vi "Fit Sinusoidal Gain.vi"(4 "Trace Select":i32 min=0 max=1000, 6 "reference 4":refnum<vi>, 7 "Cluster in":T1={"Impulse Positions"=[], "Data File"={"Data Channels"=[], "Sample Rate"=0, "Channel List"=[]}, "desaccading parameters"={"Tolerance"=0, "Acc Range"=0.0, "Sample Rate"=0, "Impulse Plane 2"=enum."Other", "Impulse dir"=FALSE}, "Stimulus"=[], "Response"=[], "Fitted Curves"=[], "Sinusoidal Fit Controls"={"Sinusoidal Response"={"Offset"=0.0, "Gain"=0.0, "Phase"=0.0, "Freq"=0.0}, "Sinusoidal Stimulus"={"Offset"=-0.1762531244084861, "Gain"=54.01231242273056, "Phase"=48.997269246957444, "Freq"=8.0}, "Stimulus\nFrequency"=8.0, "Stat."=enum."Ind. Traces", "Use Values Above to Calculate Gains"=FALSE, "Automatically Calculate \nStimulus Frequency"=FALSE, "Gain and Phase"={"Gain"=0.0, "Gain SD"=0.0, "Phase"=0.0, "Phase SD"=0.0}}, "Transient Gains"={"Line Fit Response"={"Offset"=0.0, "Slope"=0.0}, "Stimulus Equation"="", "Reponse Equation"="", "Gv"=0.0, "Ga"=0.0, "Line Fit Stimulus"={"Offset"=0.0, "Slope"=0.0}, "Ga Window (early)"=0, "Gv Window"=0, "Latency (ms)"=0.0, "Stim.Onset"=0.0, "TH/#SDs 2"=0.0, "Response Onset"=0.0, "Snap Cursor"=0, "Latency"=0, "Poly. Window"=0, "Ord."=0, "BIC"=0.0, "Poly Equation"="", "Gv SD"=0.0, "Ga SD"=0.0, "Ga Stat."=0, "Mirror"=FALSE, "MSE"=0.0, "Gv Stat."=0, "Ga 2"=0.0, "Ga SD 2"=0.0, "Ga Window  (late)"=0, "Ga Stat. 2"=0, "GV desaccading"=FALSE, "GA2 desaccading"=FALSE, "GA1 desaccading"=FALSE, "Line Fit Response 2"={"Offset"=0.0, "Slope"=0.0}, "Stimulus Equation 2"="", "Reponse Equation 2"="", "Line Fit Stimulus 2"={"Offset"=0.0, "Slope"=0.0}, "Show Line Fit Parameters "=FALSE, "Gv Line Fit Stimulus"={"Offset"=0.0, "Slope"=0.0}, "Gv Line Fit Response"={"Offset"=0.0, "Slope"=0.0}, "Latency window"=0, "Latency Stat."=0, "Line Fit Res Latency"={"Offset"=0.0, "Slope"=0.0}, "Stim Eq Latency"="", "Resp Eq Latency"="", "Line Fit Stim Latency"={"Offset"=0.0, "Slope"=0.0}, "GA Line active"=0}, "Gv Line Fit Stimulus"={"Offset"=0.0, "Slope"=0.0}, "Gv Line Fit Response"={"Offset"=0.0, "Slope"=0.0}, "Fit Calculated"=FALSE, "Excel"={"Excel._Application"=refnum, "Use Excel"=FALSE, "Worksheet SINE"=refnum, "Row SINE"=0, "Worksheet TRANS"=refnum, "Row TRANS"=0}, "desacc "={"Threshold 1 [Acc]"=0.0, "Threshold 2 [% of TH1]"=0, "tolerance"=0, "Search WD "=0.0, " always use TH2"=FALSE, "Range"=0.0, "Max time"=0.0, "Min time"=0.0, "Velocity Threshold"=0}, "Impulse Data"=refnum, "Impulse Manager"=refnum, "Graph Manager"=refnum, "Sine Fit"=[], "Excel Logger"=refnum, "Halfwave Fit Display"=refnum, "Mean Fit"=refnum} {"Sinusoidal Fit Controls"."Gain and Phase"."Phase SD" format="%.1f"; "Sinusoidal Fit Controls"."Gain and Phase"."Phase" format="%.1f"; "Sinusoidal Fit Controls"."Gain and Phase"."Gain SD" format="%.2f"; "Sinusoidal Fit Controls"."Gain and Phase"."Gain" format="%.2f"; "Sinusoidal Fit Controls"."Stimulus\nFrequency" format="%.2f"; "Sinusoidal Fit Controls"."Sinusoidal Stimulus"."Freq" format="%#.2f"; "Sinusoidal Fit Controls"."Sinusoidal Stimulus"."Offset" format="%.3f"; "Sinusoidal Fit Controls"."Sinusoidal Stimulus"."Gain" format="%.2f"; "Sinusoidal Fit Controls"."Sinusoidal Stimulus"."Phase" format="%.1f"; "Sinusoidal Fit Controls"."Sinusoidal Response"."Freq" format="%#.2f"; "Sinusoidal Fit Controls"."Sinusoidal Response"."Offset" format="%.3f"; "Sinusoidal Fit Controls"."Sinusoidal Response"."Gain" format="%.2f"; "Sinusoidal Fit Controls"."Sinusoidal Response"."Phase" format="%.1f"}, 9 "reference 3":refnum<vi>, 10 "reference in":refnum<vi>, 11 "Array in":refnum<vi>) -> (3 "Cluster out":T1={"Impulse Positions"=[], "Data File"={"Data Channels"=[], "Sample Rate"=0, "Channel List"=[]}, "desaccading parameters"={"Tolerance"=0, "Acc Range"=0.0, "Sample Rate"=0, "Impulse Plane 2"=enum."Other", "Impulse dir"=FALSE}, "Stimulus"=[], "Response"=[], "Fitted Curves"=[], "Sinusoidal Fit Controls"={"Sinusoidal Response"={"Offset"=0.0, "Gain"=0.0, "Phase"=0.0, "Freq"=0.0}, "Sinusoidal Stimulus"={"Offset"=-0.1762531244084861, "Gain"=54.01231242273056, "Phase"=48.997269246957444, "Freq"=8.0}, "Stimulus\nFrequency"=8.0, "Stat."=enum."Ind. Traces", "Use Values Above to Calculate Gains"=FALSE, "Automatically Calculate \nStimulus Frequency"=FALSE, "Gain and Phase"={"Gain"=0.0, "Gain SD"=0.0, "Phase"=0.0, "Phase SD"=0.0}}, "Transient Gains"={"Line Fit Response"={"Offset"=0.0, "Slope"=0.0}, "Stimulus Equation"="", "Reponse Equation"="", "Gv"=0.0, "Ga"=0.0, "Line Fit Stimulus"={"Offset"=0.0, "Slope"=0.0}, "Ga Window (early)"=0, "Gv Window"=0, "Latency (ms)"=0.0, "Stim.Onset"=0.0, "TH/#SDs 2"=0.0, "Response Onset"=0.0, "Snap Cursor"=0, "Latency"=0, "Poly. Window"=0, "Ord."=0, "BIC"=0.0, "Poly Equation"="", "Gv SD"=0.0, "Ga SD"=0.0, "Ga Stat."=0, "Mirror"=FALSE, "MSE"=0.0, "Gv Stat."=0, "Ga 2"=0.0, "Ga SD 2"=0.0, "Ga Window  (late)"=0, "Ga Stat. 2"=0, "GV desaccading"=FALSE, "GA2 desaccading"=FALSE, "GA1 desaccading"=FALSE, "Line Fit Response 2"={"Offset"=0.0, "Slope"=0.0}, "Stimulus Equation 2"="", "Reponse Equation 2"="", "Line Fit Stimulus 2"={"Offset"=0.0, "Slope"=0.0}, "Show Line Fit Parameters "=FALSE, "Gv Line Fit Stimulus"={"Offset"=0.0, "Slope"=0.0}, "Gv Line Fit Response"={"Offset"=0.0, "Slope"=0.0}, "Latency window"=0, "Latency Stat."=0, "Line Fit Res Latency"={"Offset"=0.0, "Slope"=0.0}, "Stim Eq Latency"="", "Resp Eq Latency"="", "Line Fit Stim Latency"={"Offset"=0.0, "Slope"=0.0}, "GA Line active"=0}, "Gv Line Fit Stimulus"={"Offset"=0.0, "Slope"=0.0}, "Gv Line Fit Response"={"Offset"=0.0, "Slope"=0.0}, "Fit Calculated"=FALSE, "Excel"={"Excel._Application"=refnum, "Use Excel"=FALSE, "Worksheet SINE"=refnum, "Row SINE"=0, "Worksheet TRANS"=refnum, "Row TRANS"=0}, "desacc "={"Threshold 1 [Acc]"=0.0, "Threshold 2 [% of TH1]"=0, "tolerance"=0, "Search WD "=0.0, " always use TH2"=FALSE, "Range"=0.0, "Max time"=0.0, "Min time"=0.0, "Velocity Threshold"=0}, "Impulse Data"=refnum, "Impulse Manager"=refnum, "Graph Manager"=refnum, "Sine Fit"=[], "Excel Logger"=refnum, "Halfwave Fit Display"=refnum, "Mean Fit"=refnum} {"Sinusoidal Fit Controls"."Gain and Phase"."Phase SD" format="%.1f"; "Sinusoidal Fit Controls"."Gain and Phase"."Phase" format="%.1f"; "Sinusoidal Fit Controls"."Gain and Phase"."Gain SD" format="%.2f"; "Sinusoidal Fit Controls"."Gain and Phase"."Gain" format="%.2f"; "Sinusoidal Fit Controls"."Stimulus\nFrequency" format="%.2f"; "Sinusoidal Fit Controls"."Sinusoidal Stimulus"."Freq" format="%#.2f"; "Sinusoidal Fit Controls"."Sinusoidal Stimulus"."Offset" format="%.3f"; "Sinusoidal Fit Controls"."Sinusoidal Stimulus"."Gain" format="%.2f"; "Sinusoidal Fit Controls"."Sinusoidal Stimulus"."Phase" format="%.1f"; "Sinusoidal Fit Controls"."Sinusoidal Response"."Freq" format="%#.2f"; "Sinusoidal Fit Controls"."Sinusoidal Response"."Offset" format="%.3f"; "Sinusoidal Fit Controls"."Sinusoidal Response"."Gain" format="%.2f"; "Sinusoidal Fit Controls"."Sinusoidal Response"."Phase" format="%.1f"})   [LabVIEW 2013]
uses:
  comm/nan operations/nan operations.lvlib
  <vilib>/Analysis/NI_AALPro.lvlib
  comm/impulse/impulse functions.lvlib
  comm/stats/stats.lvlib
  <vilib>/Analysis/NI_AALBase.lvlib
  <vilib>/Analysis/baseanly.llb/Mean (DBL).vi
  <vilib>/Analysis/1siggen.llb/Ramp Pattern by Samples.vi
  core/Classes/Sinusoidal Fit/Sinusoidal Fit.lvclass
  Polimorphic Gain and Phase VIs/Cluster Gain and Phase.vi
  Polimorphic Gain and Phase VIs/Mean Gain and Phase.vi
  Typedef_StatisticType.ctl
  Typedef - Gain and Phase.ctl
  Typedef - Sinusoidal Fit Coefficients.ctl
  Typedef - Data Analyser Main Cluster.ctl
  Typedef - Sinusoidal Fit Controls.ctl
  core/Classes/Impulse Data/Impulse Data.lvclass
  core/Classes/Impulse Manager/Impulse Manager.lvclass
  core/Classes/Impulse Data/Instance handle.ctl
  core/Classes/Graph Manager/Graph Manager.lvclass
  core/Classes/Excel Logger/Excel Logger.lvclass
  core/Classes/Fit Displays/Halfwave Fit Display/Halfwave Fit Display.lvclass
  core/Classes/Mean Fit/Mean Fit.lvclass
panel:
  # "Gain:"
  # "+/-"
  # "Phase:"
  # "+/-"
  # "Gain:"
  # "+/-"
  # "Phase:"
  # "+/-"
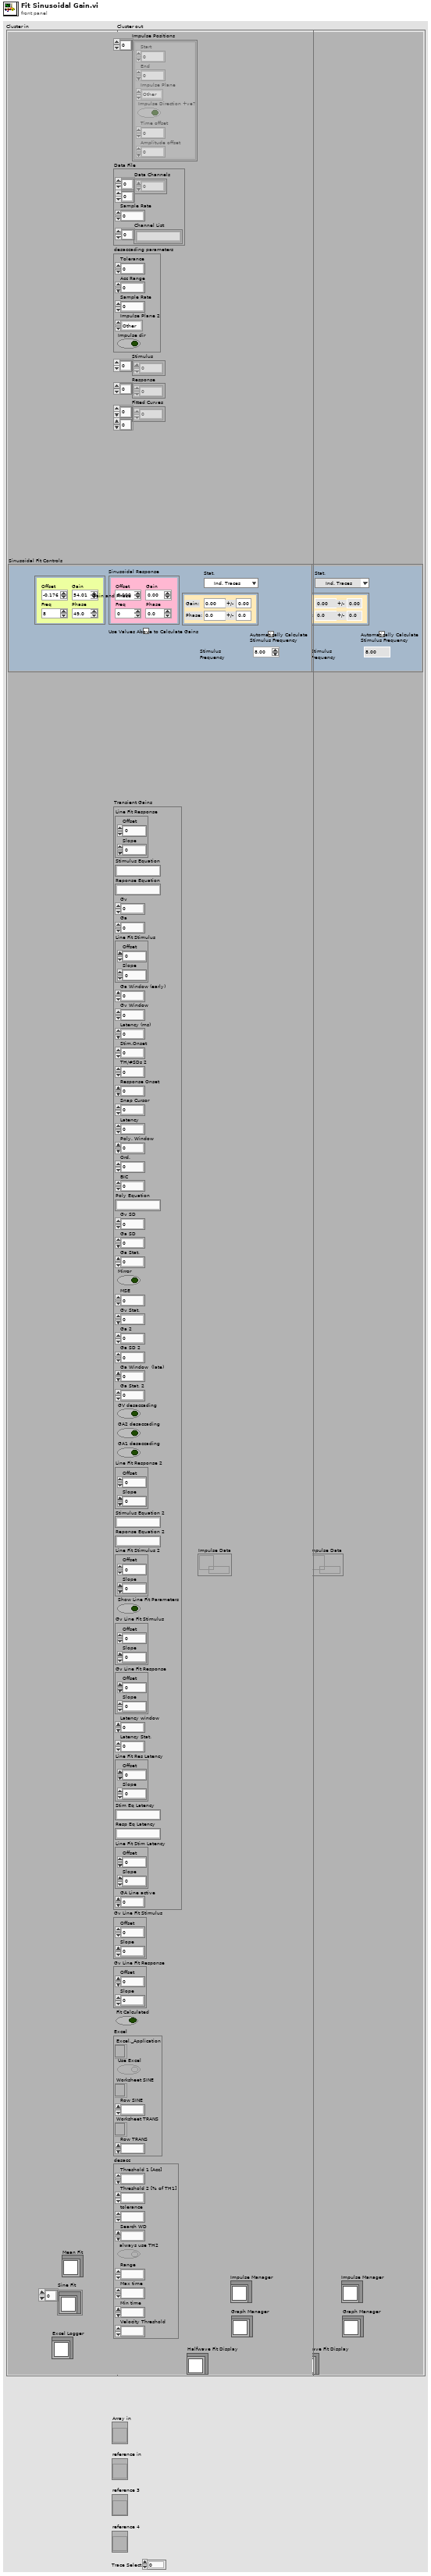
[diagram p1: front panel]
types:
  T1 = typedef "Typedef - Data Analyser Main Cluster.ctl" = cluster{"Impulse Positions":cluster{"Start":i32, "End":i32, "Impulse Plane":enum16{"Other", "Yaw", "Pitch", "Roll", "LARP", "RALP"}, "Impulse Direction +ve?":bool, "Time offset":i32, "Amplitude offset":dbl}[], "Data File":cluster{"Data Channels":dbl[][], "Sample Rate":i32, "Channel List":string[]}, "desaccading parameters":cluster{"Tolerance":i32, "Acc Range":dbl, "Sample Rate":i32, "Impulse Plane 2":enum16{"Other", "Yaw", "Pitch", "Roll", "LARP", "RALP"}, "Impulse dir":bool}, "Stimulus":dbl[], "Response":dbl[], "Fitted Curves":dbl[][], "Sinusoidal Fit Controls":T2, "Transient Gains":cluster{"Line Fit Response":cluster{"Offset":dbl, "Slope":dbl}, "Stimulus Equation":string, "Reponse Equation":string, "Gv":dbl, "Ga":dbl, "Line Fit Stimulus":cluster{"Offset":dbl, "Slope":dbl}, "Ga Window (early)":u16, "Gv Window":u16, "Latency (ms)":dbl, "Stim.Onset":dbl, "TH/#SDs 2":dbl, "Response Onset":dbl, "Snap Cursor":u16, "Latency":u16, "Poly. Window":u16, "Ord.":i32, "BIC":dbl, "Poly Equation":string, "Gv SD":dbl, "Ga SD":dbl, "Ga Stat.":u16, "Mirror":bool, "MSE":dbl, "Gv Stat.":u16, "Ga 2":dbl, "Ga SD 2":dbl, "Ga Window  (late)":u16, "Ga Stat. 2":u16, "GV desaccading":bool, "GA2 desaccading":bool, "GA1 desaccading":bool, "Line Fit Response 2":cluster{"Offset":dbl, "Slope":dbl}, "Stimulus Equation 2":string, "Reponse Equation 2":string, "Line Fit Stimulus 2":cluster{"Offset":dbl, "Slope":dbl}, "Show Line Fit Parameters ":bool, "Gv Line Fit Stimulus":cluster{"Offset":dbl, "Slope":dbl}, "Gv Line Fit Response":cluster{"Offset":dbl, "Slope":dbl}, "Latency window":u16, "Latency Stat.":u16, "Line Fit Res Latency":cluster{"Offset":dbl, "Slope":dbl}, "Stim Eq Latency":string, "Resp Eq Latency":string, "Line Fit Stim Latency":cluster{"Offset":dbl, "Slope":dbl}, "GA Line active":i32}, "Gv Line Fit Stimulus":cluster{"Offset":dbl, "Slope":dbl}, "Gv Line Fit Response":cluster{"Offset":dbl, "Slope":dbl}, "Fit Calculated":bool, "Excel":cluster{"Excel._Application":refnum<k7>, "Use Excel":bool, "Worksheet SINE":refnum<k7>, "Row SINE":i32, "Worksheet TRANS":refnum<k7>, "Row TRANS":i32}, "desacc ":cluster{"Threshold 1 [Acc]":dbl, "Threshold 2 [% of TH1]":i32, "tolerance":i32, "Search WD ":dbl, " always use TH2":bool, "Range":dbl, "Max time":dbl, "Min time":dbl, "Velocity Threshold":i32}, "Impulse Data":T6, "Impulse Manager":refnum<class "Impulse Manager.lvclass">, "Graph Manager":refnum<class "Graph Manager.lvclass">, "Sine Fit":refnum<class "Sinusoidal Fit.lvclass">[], "Excel Logger":refnum<class "Excel Logger.lvclass">, "Halfwave Fit Display":refnum<class "Halfwave Fit Display.lvclass">, "Mean Fit":refnum<class "Mean Fit.lvclass">}
  T2 = typedef "Typedef - Sinusoidal Fit Controls.ctl" = cluster{"Sinusoidal Response":T3, "Sinusoidal Stimulus":T3, "Stimulus\nFrequency":dbl, "Stat.":T4, "Use Values Above to Calculate Gains":bool, "Automatically Calculate \nStimulus Frequency":bool, "Gain and Phase":T5}
  T3 = typedef "Typedef - Sinusoidal Fit Coefficients.ctl" = cluster{"Offset":dbl, "Gain":dbl, "Phase":dbl, "Freq":dbl}
  T4 = typedef "Typedef_StatisticType.ctl" = enum16{"Mean Trace", "Ind. Traces"}
  T5 = typedef "Typedef - Gain and Phase.ctl" = cluster{"Gain":dbl, "Gain SD":dbl, "Phase":dbl, "Phase SD":dbl}
  T6 = typedef "Impulse Data.lvclass/Instance handle.ctl" = refnum<data-value>
  T7 = cluster{"Data Channels":dbl[][], "Sample Rate":i32, "Channel List":string[]}
  T8 = cluster{"Start":i32, "End":i32, "Impulse Plane":enum16{"Other", "Yaw", "Pitch", "Roll", "LARP", "RALP"}, "Impulse Direction +ve?":bool, "Time offset":i32, "Amplitude offset":dbl}[]
  T9 = enum16{"Other", "Yaw", "Pitch", "Roll", "LARP", "RALP"}
  T10 = cluster{"Threshold 1 [Acc]":dbl, "Threshold 2 [% of TH1]":i32, "tolerance":i32, "Search WD ":dbl, " always use TH2":bool, "Range":dbl, "Max time":dbl, "Min time":dbl, "Velocity Threshold":i32}
  T11 = typedef "core.lvlib/TD_Impulse Parameter.ctl" = cluster{"Color Box":u32, "Boolean":bool, "List 2":u16, "Boolean 2":bool, "Boolean 3":bool, "Offset":dbl, "Gain":dbl}[]
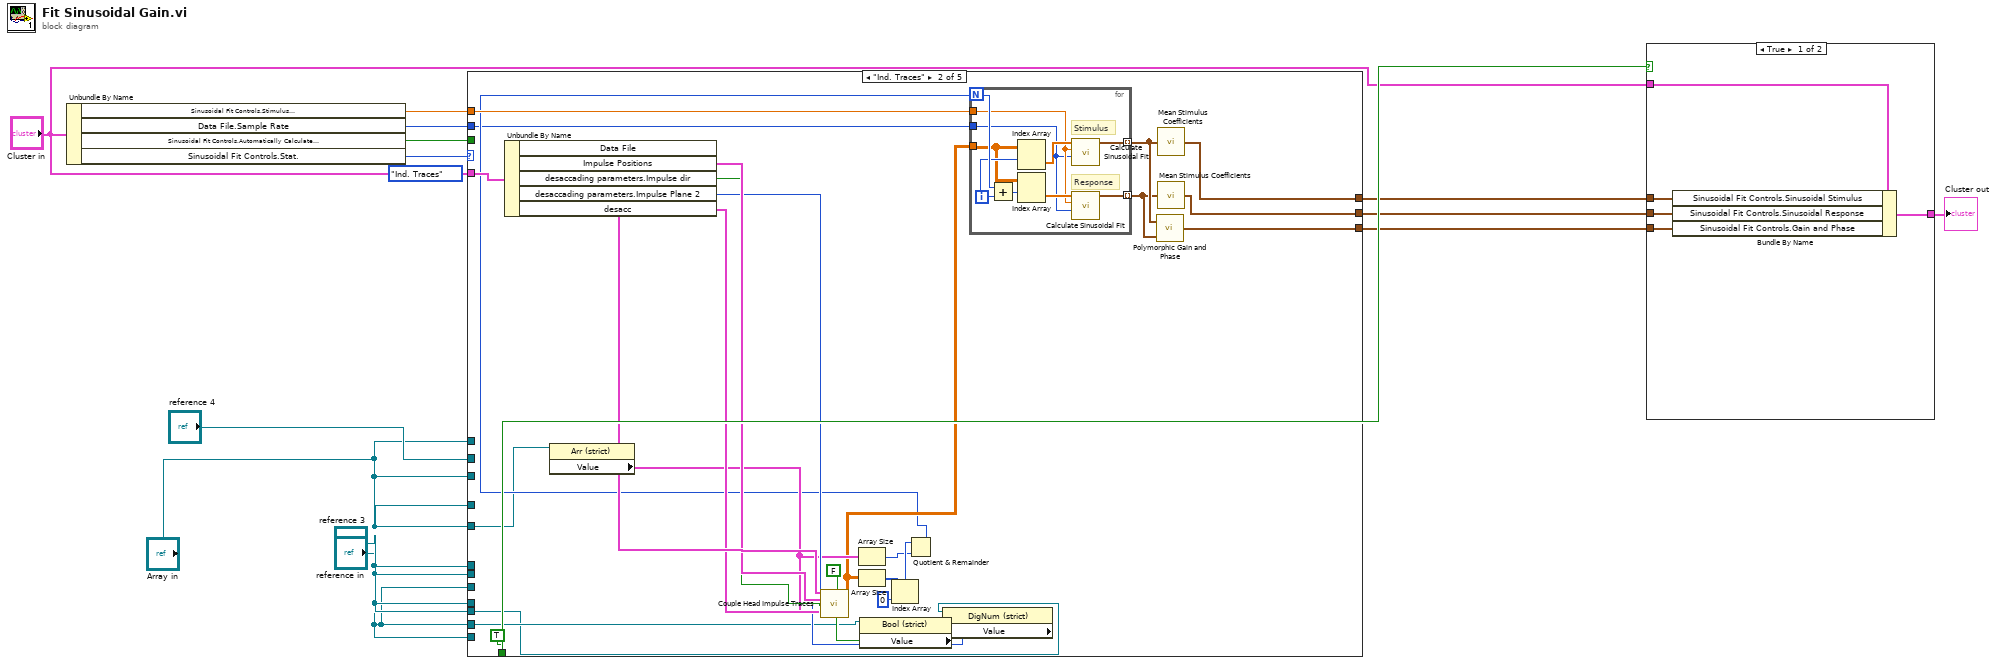
[diagram p0: block diagram]
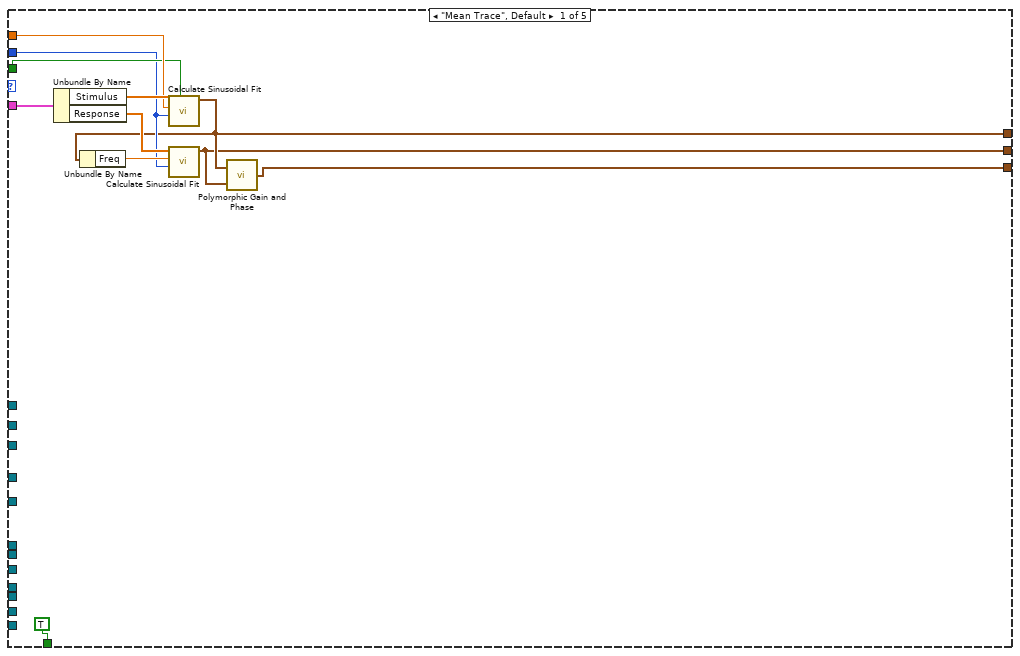
[diagram p2: hidden frame]
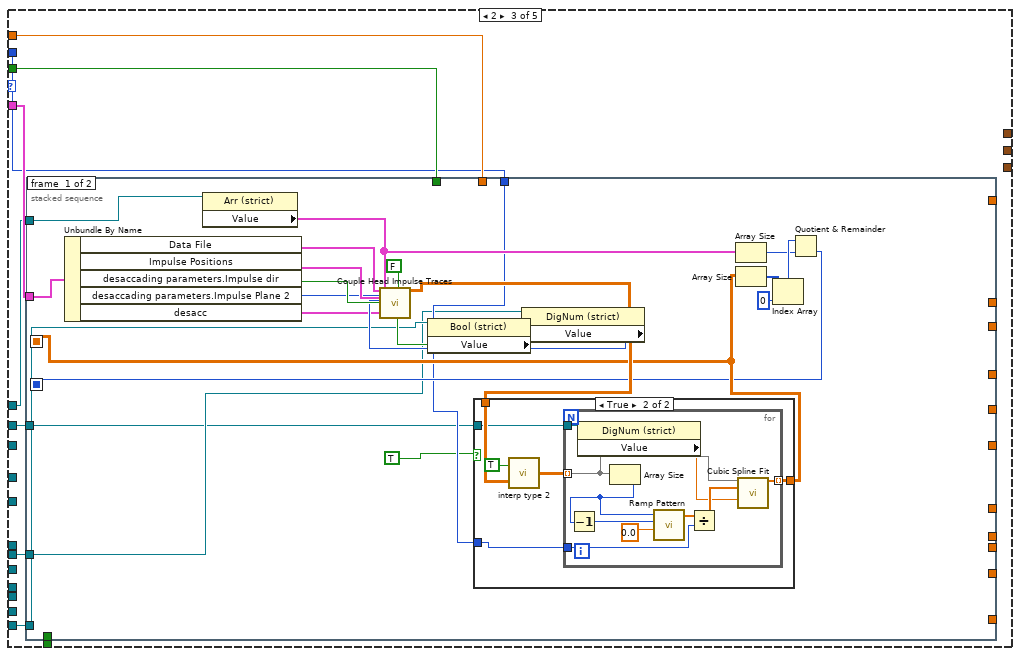
[diagram p3: hidden frame]
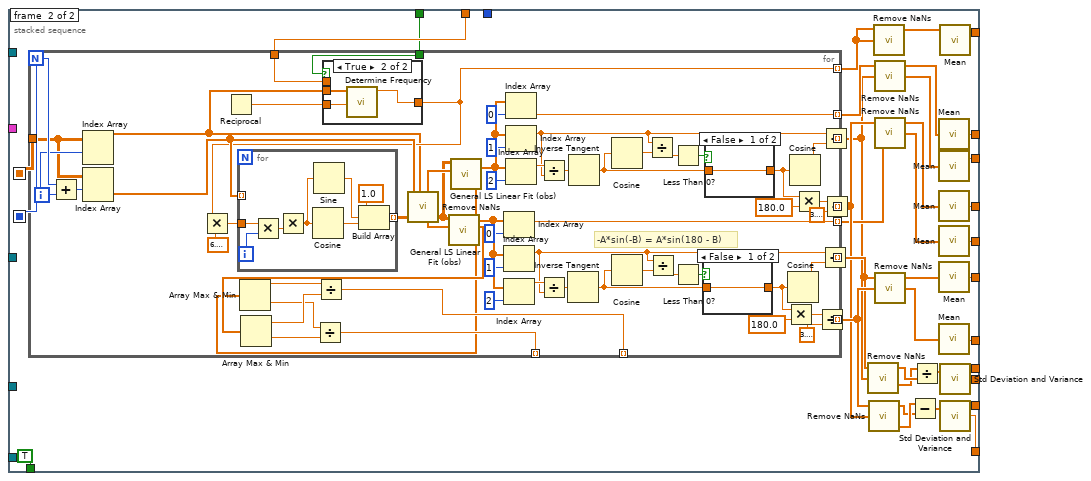
[diagram p5: hidden frame]
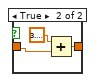
[diagram p7: hidden frame]
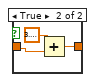
[diagram p8: hidden frame]
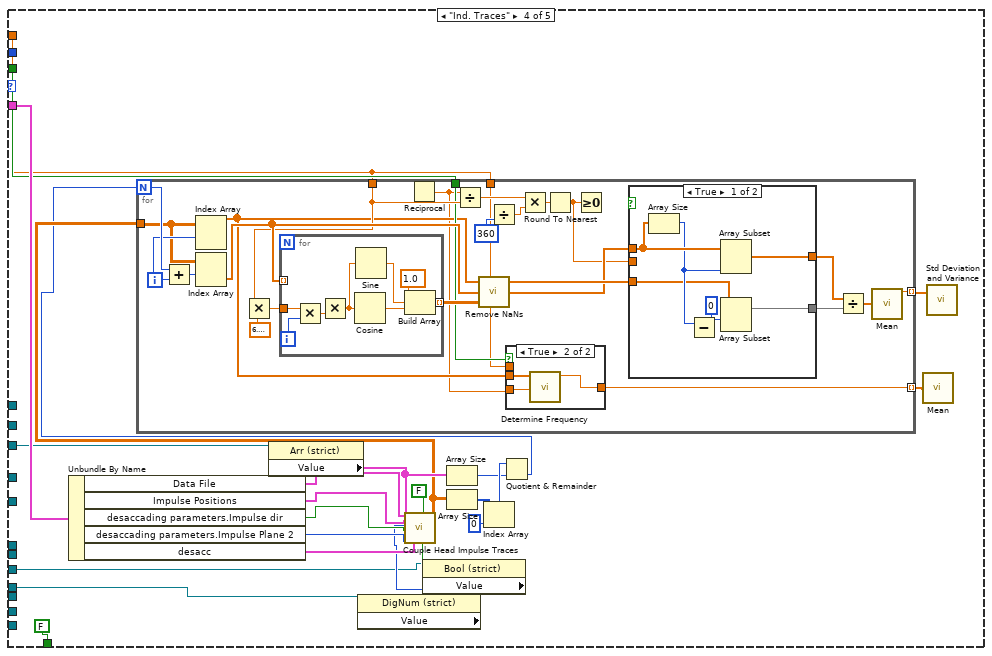
[diagram p9: hidden frame]
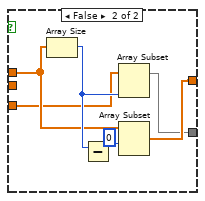
[diagram p11: hidden frame]
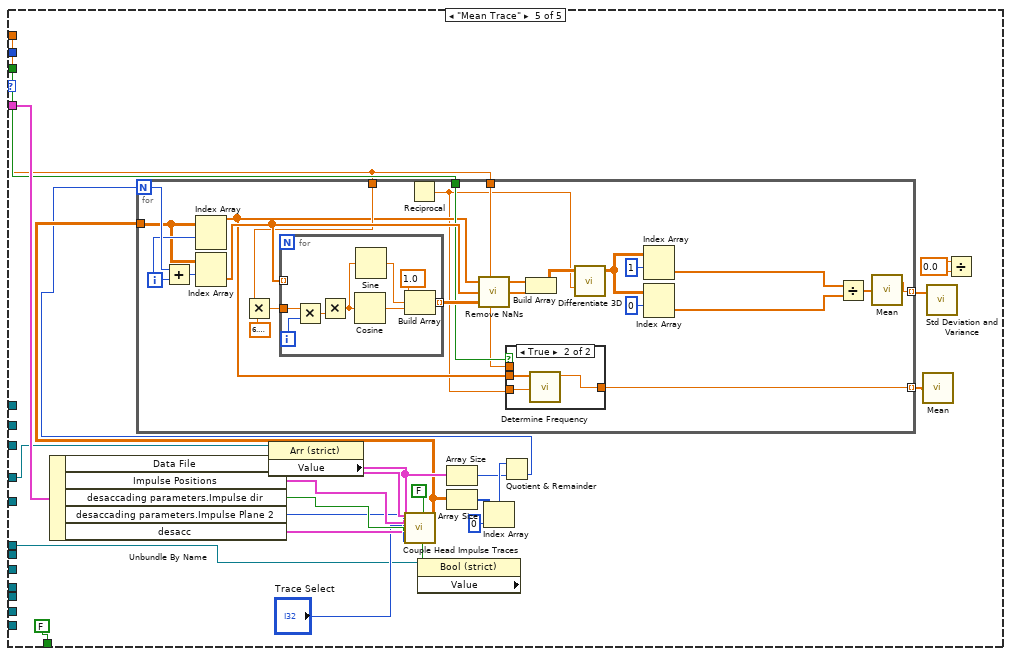
[diagram p12: hidden frame]
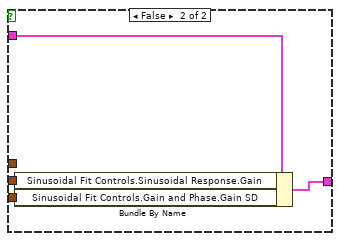
[diagram p14: hidden frame]
diagram:
  (unwired) Typedef_StatisticType."Ind. Traces" ("Sinusoidal Fit Controls.Stat.")
  n1 = Unbundle By Name("Cluster in") -> ("Sinusoidal Fit Controls.Stimulus\nFrequency"=w13:dbl, "Data File.Sample Rate"=w1:i32, "Sinusoidal Fit Controls.Automatically Calculate \nStimulus Frequency"=w14:bool, "Sinusoidal Fit Controls.Stat."=w10:T4)
  n2 = case shown="\"Ind. Traces\"" w10 {
    tunnel: w13 -> [w22 w52 w71 w236 w308]
    tunnel: "Cluster in" -> [w25 w40 w68 w242 w315]
    tunnel: [TRUE TRUE w70 FALSE FALSE] -> w12
    tunnel: w14 -> [w21 _ w69 w237 w309]
    tunnel: w1 -> [w18 w31 w67 _ _]
    tunnel: "Array in" -> [_ w34 _ _ _]
    tunnel: "reference in" -> [_ w33 _ _ _]
    tunnel: "reference 3" -> [_ w32 _ _ _]
    tunnel: "Array in" -> [_ _ w66 _ _]
    tunnel: "reference in" -> [_ _ w65 _ _]
    tunnel: "reference 3" -> [_ _ w64 _ _]
    tunnel: "reference 4" -> [_ _ w63 _ _]
    tunnel: "Array in" -> [_ _ _ w232 _]
    tunnel: "reference in" -> [_ _ _ w231 _]
    tunnel: "reference 3" -> [_ _ _ w230 _]
    tunnel: "Array in" -> [_ _ _ _ w304]
    tunnel: "reference in" -> [_ _ _ _ w303]
    tunnel: [w17 w30 _ _ _] -> w4
    tunnel: [w16 w29 _ _ _] -> w3
    tunnel: [w15 w26 _ _ _] -> w2
    frame "Mean Trace", Default {
      n3 = Unbundle By Name(w25) -> ("Stimulus"=w23:dbl[], "Response"=w19:dbl[])
      n4 = call "Calculate Sinusoidal Fit.vi"(7:w21, "Sample Rate"=w18, "Stimulus\nFrequency"=w22, "Data in"=w23) -> ("Coefficients"=w17:T3)  [unwired: 6 in, 1 out]
      n5 = Unbundle By Name(w17) -> ("Freq"=w20:dbl)
      n6 = call "Calculate Sinusoidal Fit.vi"("Sample Rate"=w18, "Stimulus\nFrequency"=w20, "Data in"=w19) -> ("Coefficients"=w16:T3)  [unwired: 7 in, 1 out]
      n7 = call-poly "Polymorphic Gain and Phase.vi"("Response"=w16, "Stimulus"=w17) -> ("Gain and Phase out"=w15:T5)
    }
    frame "Ind. Traces" {
      n8 = Unbundle By Name(w40) -> ("Data File"=w51:T7, "Impulse Positions"=w50:T8, "desaccading parameters.Impulse dir"=w49:bool, "desaccading parameters.Impulse Plane 2"=w48:T9, "desacc"=w47:T10)
      n9 = property class="Arr (strict)"(reference=w34) -> ("Value"=w45:T11)  [unwired: 1 in, 2 out]
      n10 = Array Size(array=w45) -> (size(s)=w41:i32)
      n11 = property class="Bool (strict)"(reference=w33) -> ("Value"=w36:bool)  [unwired: 1 in, 2 out]
      n12 = property class="DigNum (strict)"(reference=w32) -> ("Value"=w35:i32)  [unwired: 1 in, 2 out]
      n13 = call "Couple Head Impulse Traces.vi"("Data Input"=w51, "Impulse Positions"=w50, "Trace Select"=w35, "Impulse Direction +ve?"=w49, "Impulse Plane"=w48, "Mean and STD"=FALSE ("Mean Traces"), "Plot Selection 2"=w45, "desacc"=w47, "Interpolate"=w36) -> ("Impulses"=w39:dbl[][])  [unwired: 7 in, 3 out]
      n14 = Array Size(array=w39) -> (size(s)=w44:i32[])
      n15 = Index Array(array=w44, index=0) -> (element=w42:i32)
      n16 = Quotient & Remainder(x=w42, y=w41) -> (floor(x/y)=w38:i32)  [unwired: 1 out]
      n17 = for {
        N: w38 -> [w61]
        tunnel: w52 -> [w56]
        tunnel: w39 -> [w59]
        tunnel: w31 -> [w55]
        tunnel: [w54] -> w27 mode=indexing
        tunnel: [w53] -> w28 mode=indexing
        i -> [w60]
        # "Response"
        # "Stimulus"
        n18 = Add(x=w61, y=w60) -> (x+y=w62:i32)
        n19 = Index Array(array=w59, index (row)=w60) -> (element=w58:dbl[])  [unwired: 1 in]
        n20 = Index Array(array=w59, index (row)=w62) -> (element=w57:dbl[])  [unwired: 1 in]
        n21 = call "Calculate Sinusoidal Fit.vi"("Sample Rate"=w55, "Stimulus\nFrequency"=w56, "Data in"=w58) -> ("Coefficients"=w53:T3)  [unwired: 7 in, 1 out]
        n22 = call "Calculate Sinusoidal Fit.vi"("Sample Rate"=w55, "Stimulus\nFrequency"=w56, "Data in"=w57) -> ("Coefficients"=w54:T3)  [unwired: 7 in, 1 out]
      }
      n23 = call-poly "Polymorphic Gain and Phase.vi"("Response"=w27, "Stimulus"=w28) -> ("Gain and Phase out"=w26:T5)
      n24 = call "Mean Stimulus Coefficients.vi"("Coefficients in"=w28) -> ("Mean Coefficients out"=w30:T3)
      n25 = call "Mean Stimulus Coefficients.vi"("Coefficients in"=w27) -> ("Mean Coefficients out"=w29:T3)
    }
    frame 2 {
      n26 = stacked-sequence {
        seq-local: [w79 _] -> [_ w113]
        seq-local: [w78 _] -> [_ w112]
        tunnel: w71 -> [_ w147]
        tunnel: [_ w146] -> _
        tunnel: [_ w145] -> _
        tunnel: [_ w144] -> _
        tunnel: [_ w143] -> _
        tunnel: [_ w142] -> _
        tunnel: [_ w141] -> _
        tunnel: [_ w139] -> _
        tunnel: [_ w137] -> _
        tunnel: [_ w136] -> _
        tunnel: [_ w135] -> _
        tunnel: [_ TRUE] -> w70
        tunnel: w69 -> [_ w117]
        tunnel: [_ w114] -> _
        tunnel: w68 -> [w83 _]
        tunnel: w67 -> [w77 _]
        tunnel: w66 -> [w75 _]
        tunnel: w65 -> [w74 _]
        tunnel: w64 -> [w73 _]
        tunnel: w63 -> [w72 _]
        frame #0 {
          n27 = Unbundle By Name(w83) -> ("Data File"=w94:T7, "Impulse Positions"=w93:T8, "desaccading parameters.Impulse dir"=w92:bool, "desaccading parameters.Impulse Plane 2"=w91:T9, "desacc"=w81:T10)
          n28 = property class="Arr (strict)"(reference=w75) -> ("Value"=w89:T11)  [unwired: 1 in, 2 out]
          n29 = property class="Bool (strict)"(reference=w74) -> ("Value"=w84:bool)  [unwired: 1 in, 2 out]
          n30 = property class="DigNum (strict)"(reference=w73) -> ("Value"=w82:i32)  [unwired: 1 in, 2 out]
          n31 = call "Couple Head Impulse Traces.vi"("Data Input"=w94, "Impulse Positions"=w93, "Trace Select"=w82, "Impulse Direction +ve?"=w92, "Impulse Plane"=w91, "Mean and STD"=FALSE ("Mean Traces"), "Plot Selection 2"=w89, "desacc"=w81, "Interpolate"=w84) -> ("Impulses"=w80:dbl[][])  [unwired: 7 in, 3 out]
          n32 = case shown="True" TRUE {
            tunnel: w80 -> [w95 w100]
            tunnel: [w95 w101] -> w79
            tunnel: w77 -> [_ w98]
            tunnel: w72 -> [_ w96]
            frame False {
            }
            frame True {
              n33 = call "interp type 2.vi"("NaN"=w100, "Remove front and end"=TRUE) -> ("Interpolated"=w99:dbl[][])
              n34 = for {
                tunnel: w98 -> [w105]
                tunnel: w99 -> [w108] mode=indexing
                tunnel: [w107] -> w101 mode=indexing
                tunnel: w96 -> [w102]
                n35 = property class="DigNum (strict)"(reference=w102) -> ("Value"=w103:dbl)  [unwired: 1 in, 2 out]
                n36 = Array Size(array=w108) -> (size(s)=w110:i32)
                n37 = Decrement(x=w110) -> (x-1=w109:i32)
                n38 = call-poly <vilib>:"Ramp Pattern.vi"("start"=0.0, "end"=w109, "samples"=w110) -> ("Ramp Pattern"=w106:dbl[])  [unwired: 7 in, 1 out]
                n39 = Divide(x=w106, y=w105) -> (x/y=w104:dbl[])
                n40 = call <vilib>:"Cubic Spline Fit.vi"("Y"=w108, "X"=w104, "balance parameter"=w103) -> ("Best Cubic Spline Fit"=w107:dbl[])  [unwired: 11 in, 1 out]
              }
            }
          }
          n41 = Array Size(array=w89) -> (size(s)=w85:i32)
          n42 = Array Size(array=w79) -> (size(s)=w88:i32[])
          n43 = Index Array(array=w88, index=0) -> (element=w86:i32)
          n44 = Quotient & Remainder(x=w86, y=w85) -> (floor(x/y)=w78:i32)  [unwired: 1 out]
        }
        frame #1 {
          n45 = for {
            N: w112 -> [w164]
            tunnel: [w172] -> w123 mode=indexing
            tunnel: [w171] -> w127 mode=indexing
            tunnel: [w170] -> w121 mode=indexing
            tunnel: [w168] -> w125 mode=indexing
            tunnel: [w167] -> w129 mode=indexing
            tunnel: [w166] -> w132 mode=indexing
            tunnel: w147 -> [w159]
            tunnel: w113 -> [w162]
            tunnel: w117 -> [w160]
            tunnel: [w158] -> w116 mode=indexing
            tunnel: [w151] -> _ mode=indexing
            tunnel: [w150] -> _ mode=indexing
            i -> [w163]
            # "-A*sin(-B) = A*sin(180 - B)"
            n46 = Add(x=w164, y=w163) -> (x+y=w165:i32)
            n47 = Index Array(array=w162, index (row)=w163) -> (element=w157:dbl[])  [unwired: 1 in]
            n48 = Index Array(array=w162, index (row)=w165) -> (element=w161:dbl[])  [unwired: 1 in]
            n49 = Reciprocal() -> (1/x=w156:dbl)  [unwired: 1 in]
            n50 = case shown="True" w160 {
              tunnel: [w210 w211] -> w158
              tunnel: w159 -> [w210 _]
              tunnel: w157 -> [_ w213]
              tunnel: w156 -> [_ w212]
              frame False {
              }
              frame True {
                n51 = call "Determine Frequency.vi"("Sample Rate"=w212, "Signal (in)"=w213) -> ("Fundamental frequency"=w211:dbl)  [unwired: 5 in]
              }
            }
            n52 = Multiply(x=w158, y=6.283185307179586) -> (x*y=w169:dbl)
            n53 = for {
              tunnel: w169 -> [w229]
              tunnel: [w222] -> w175 mode=indexing
              tunnel: w161 -> [_] mode=indexing
              i -> [w228]
              n54 = Multiply(x=w229, y=w228) -> (x*y=w227:dbl)
              n55 = Multiply(y=w227) -> (x*y=w226:dbl)  [unwired: 1 in]
              n56 = Cosine(x=w226) -> (cos(x)=w225:dbl)
              n57 = Sine(x=w226) -> (sin(x)=w224:dbl)
              n58 = Build Array(1.0 ("Input Element"), w224, w225) -> (w222:dbl[])
            }
            n59 = call "Remove NaNs.vi"("Sinusoid"=w175, "Response"=w161, "Stimulus"=w157) -> ("Sinusoid (out)"=w174:dbl[][], "Response (out)"=w176:dbl[], "Stimulus (out)"=w173:dbl[])
            n60 = call <vilib>:"General LS Linear Fit (obs).vi"("H"=w174, "Y"=w173) -> ("Coefficients"=w207:dbl[], "Best Fit"=w149:dbl[])  [unwired: 3 in, 3 out]
            n61 = Array Max & Min(array=w149) -> (max value=w154:dbl, min value=w153:dbl)  [unwired: 2 out]
            n62 = call <vilib>:"General LS Linear Fit (obs).vi"("H"=w174, "Y"=w176) -> ("Coefficients"=w208:dbl[], "Best Fit"=w148:dbl[])  [unwired: 3 in, 3 out]
            n63 = Array Max & Min(array=w148) -> (max value=w155:dbl, min value=w152:dbl)  [unwired: 2 out]
            n64 = Divide(x=w152, y=w153) -> (x/y=w151:dbl)
            n65 = Divide(x=w155, y=w154) -> (x/y=w150:dbl)
            n66 = Index Array(array=w207, index=0 ("Index")) -> (element=w168:dbl)
            n67 = Index Array(array=w207, index=1 ("Index")) -> (element=w181:dbl)
            n68 = Index Array(array=w207, index=2 ("Index")) -> (element=w199:dbl)
            n69 = Index Array(array=w208, index=0 ("Index")) -> (element=w172:dbl)
            n70 = Index Array(array=w208, index=1 ("Index")) -> (element=w184:dbl)
            n71 = Index Array(array=w208, index=2 ("Index")) -> (element=w200:dbl)
            n72 = Divide(x=w200, y=w184) -> (x/y=w189:dbl)
            n73 = Divide(x=w199, y=w181) -> (x/y=w193:dbl)
            n74 = Inverse Tangent(1:w193) -> (0:w185:dbl)
            n75 = Inverse Tangent(1:w189) -> (0:w186:dbl)
            n76 = Cosine(x=w186) -> (cos(x)=w183:dbl)
            n77 = Cosine(x=w185) -> (cos(x)=w182:dbl)
            n78 = Divide(x=w184, y=w183) -> (x/y=w179:dbl)
            n79 = Divide(x=w181, y=w182) -> (x/y=w178:dbl)
            n80 = Less Than 0?(x=w179) -> (x < 0?=w180:bool)
            n81 = Less Than 0?(x=w178) -> (x < 0?=w177:bool)
            n82 = case shown="False" w177 {
              tunnel: w185 -> [w214 w216]
              tunnel: [w214 w215] -> w187
              frame False {
              }
              frame True {
                n83 = Add(x=3.141592653589793, y=w216) -> (x+y=w215:dbl)
              }
            }
            n84 = case shown="False" w180 {
              tunnel: w186 -> [w218 w220]
              tunnel: [w218 w219] -> w188
              frame False {
              }
              frame True {
                n85 = Add(x=3.141592653589793, y=w220) -> (x+y=w219:dbl)
              }
            }
            n86 = Multiply(x=w187, y=180.0) -> (x*y=w196:dbl)
            n87 = Cosine(x=w187) -> (cos(x)=w198:dbl)
            n88 = Cosine(x=w188) -> (cos(x)=w197:dbl)
            n89 = Multiply(x=w188, y=180.0) -> (x*y=w190:dbl)
            n90 = Divide(x=w196, y=3.141592653589793) -> (x/y=w166:dbl)
            n91 = Divide(x=w181, y=w198) -> (x/y=w167:dbl)
            n92 = Divide(x=w184, y=w197) -> (x/y=w170:dbl)
            n93 = Divide(x=w190, y=3.141592653589793) -> (x/y=w171:dbl)
          }
          n94 = call "Remove NaNs.vi"("Response"=w121, "Stimulus"=w129) -> ("Response (out)"=w133:dbl[], "Stimulus (out)"=w134:dbl[])  [unwired: 1 in, 1 out]
          n95 = call "Remove NaNs.vi"("Response"=w127, "Stimulus"=w132) -> ("Response (out)"=w120:dbl[], "Stimulus (out)"=w119:dbl[])  [unwired: 1 in, 1 out]
          n96 = call "Remove NaNs.vi"("Response"=w116, "Stimulus"=w116) -> ("Stimulus (out)"=w115:dbl[])  [unwired: 1 in, 2 out]
          n97 = call "Remove NaNs.vi"("Response"=w121, "Stimulus"=w123) -> ("Response (out)"=w122:dbl[], "Stimulus (out)"=w124:dbl[])  [unwired: 1 in, 1 out]
          n98 = call "Remove NaNs.vi"("Response"=w125, "Stimulus"=w127) -> ("Response (out)"=w126:dbl[], "Stimulus (out)"=w128:dbl[])  [unwired: 1 in, 1 out]
          n99 = call "Remove NaNs.vi"("Response"=w132, "Stimulus"=w129) -> ("Response (out)"=w131:dbl[], "Stimulus (out)"=w130:dbl[])  [unwired: 1 in, 1 out]
          n100 = Subtract(x=w120, y=w119) -> (x-y=w138:dbl[])
          n101 = Divide(x=w133, y=w134) -> (x/y=w140:dbl[])
          n102 = call-poly <vilib>:"Mean.vi"("X"=w124) -> ("mean"=w146:dbl)  [unwired: 1 out]
          n103 = call-poly <vilib>:"Mean.vi"("X"=w122) -> ("mean"=w145:dbl)  [unwired: 1 out]
          n104 = call-poly <vilib>:"Mean.vi"("X"=w128) -> ("mean"=w144:dbl)  [unwired: 1 out]
          n105 = call-poly <vilib>:"Mean.vi"("X"=w126) -> ("mean"=w143:dbl)  [unwired: 1 out]
          n106 = call-poly <vilib>:"Mean.vi"("X"=w130) -> ("mean"=w142:dbl)  [unwired: 1 out]
          n107 = call-poly <vilib>:"Mean.vi"("X"=w131) -> ("mean"=w141:dbl)  [unwired: 1 out]
          n108 = call-poly <vilib>:"Mean.vi"("X"=w115) -> ("mean"=w114:dbl)  [unwired: 1 out]
          n109 = call "Std Deviation and Variance.vi"("X"=w140) -> ("mean"=w139:dbl, "standard deviation"=w136:dbl)  [unwired: 1 in, 1 out]
          n110 = call "Std Deviation and Variance.vi"("X"=w138) -> ("mean"=w137:dbl, "standard deviation"=w135:dbl)  [unwired: 1 in, 1 out]
        }
      }
    }
    frame "Ind. Traces" {
      n111 = Unbundle By Name(w242) -> ("Data File"=w253:T7, "Impulse Positions"=w252:T8, "desaccading parameters.Impulse dir"=w251:bool, "desaccading parameters.Impulse Plane 2"=w250:T9, "desacc"=w249:T10)
      n112 = property class="Arr (strict)"(reference=w232) -> ("Value"=w247:T11)  [unwired: 1 in, 2 out]
      n113 = property class="DigNum (strict)"(reference=w230) -> ("Value"=w233:i32)  [unwired: 1 in, 2 out]
      n114 = property class="Bool (strict)"(reference=w231) -> ("Value"=w234:bool)  [unwired: 1 in, 2 out]
      n115 = call "Couple Head Impulse Traces.vi"("Data Input"=w253, "Impulse Positions"=w252, "Trace Select"=w233, "Impulse Direction +ve?"=w251, "Impulse Plane"=w250, "Mean and STD"=FALSE ("Mean Traces"), "Plot Selection 2"=w247, "desacc"=w249, "Interpolate"=w234) -> ("Impulses"=w241:dbl[][])  [unwired: 7 in, 3 out]
      n116 = Array Size(array=w247) -> (size(s)=w243:i32)
      n117 = Array Size(array=w241) -> (size(s)=w246:i32[])
      n118 = Index Array(array=w246, index=0) -> (element=w244:i32)
      n119 = Quotient & Remainder(x=w244, y=w243) -> (floor(x/y)=w240:i32)  [unwired: 1 out]
      n120 = for {
        N: w240 -> [w274]
        tunnel: [w269] -> w239 mode=indexing
        tunnel: w236 -> [w268]
        tunnel: w241 -> [w272]
        tunnel: w237 -> [w258]
        tunnel: w236 -> [w257]
        tunnel: [w254] -> w235 mode=indexing
        i -> [w273]
        n121 = Add(x=w274, y=w273) -> (x+y=w275:i32)
        n122 = Index Array(array=w272, index (row)=w273) -> (element=w256:dbl[])  [unwired: 1 in]
        n123 = Index Array(array=w272, index (row)=w275) -> (element=w271:dbl[])  [unwired: 1 in]
        n124 = Multiply(x=w268, y=6.283185307179586) -> (x*y=w276:dbl)
        n125 = for {
          tunnel: w276 -> [w302]
          tunnel: [w295] -> w277 mode=indexing
          tunnel: w271 -> [_] mode=indexing
          i -> [w301]
          n126 = Multiply(x=w302, y=w301) -> (x*y=w300:dbl)
          n127 = Multiply(y=w300) -> (x*y=w299:dbl)  [unwired: 1 in]
          n128 = Cosine(x=w299) -> (cos(x)=w298:dbl)
          n129 = Sine(x=w299) -> (sin(x)=w297:dbl)
          n130 = Build Array(1.0 ("Input Element"), w297, w298) -> (w295:dbl[])
        }
        n131 = Reciprocal() -> (1/x=w255:dbl)  [unwired: 1 in]
        n132 = Divide(x=w255, y=w268) -> (x/y=w265:dbl)
        n133 = call "Remove NaNs.vi"("Sinusoid"=w277, "Response"=w271, "Stimulus"=w256) -> ("Response (out)"=w262:dbl[], "Stimulus (out)"=w263:dbl[])  [unwired: 1 out]
        n134 = Divide(y=360) -> (x/y=w266:dbl)  [unwired: 1 in]
        n135 = case shown="True" w258 {
          tunnel: [w279 w280] -> w254
          tunnel: w257 -> [w279 _]
          tunnel: w256 -> [_ w282]
          tunnel: w255 -> [_ w281]
          frame False {
          }
          frame True {
            n136 = call "Determine Frequency.vi"("Sample Rate"=w281, "Signal (in)"=w282) -> ("Fundamental frequency"=w280:dbl)  [unwired: 5 in]
          }
        }
        n137 = Multiply(x=w265, y=w266) -> (x*y=w264:dbl)
        n138 = Round To Nearest(number=w264) -> (nearest integer value=w261:dbl)
        n139 = Greater Or Equal To 0?(x=w261) -> ()  [unwired: 1 out]
        n140 = case shown="True" {
          selector: _ -> [_ _]
          tunnel: w263 -> [w284 w291]
          tunnel: w262 -> [w288 w292]
          tunnel: w261 -> [_ _]
          tunnel: [w285 w290] -> w260
          tunnel: [w283 w289] -> w259
          frame True {
            n141 = Array Size(array=w288) -> (size(s)=w286:i32)
            n142 = Subtract(x=w286) -> ()  [unwired: 1 in, 1 out]
            n143 = Array Subset(array=w288, length=w286) -> (w285:dbl[])  [unwired: 1 in]
            n144 = Array Subset(array=w284, index=0) -> (w283:dbl[])  [unwired: 1 in]
          }
          frame False {
            n145 = Array Size(array=w292) -> (size(s)=w293:i32)
            n146 = Subtract(x=w293) -> ()  [unwired: 1 in, 1 out]
            n147 = Array Subset(array=w291, length=w293) -> (w289:dbl[])  [unwired: 1 in]
            n148 = Array Subset(array=w292, index=0) -> (w290:dbl[])  [unwired: 1 in]
          }
        }
        n149 = Divide(x=w260, y=w259) -> (x/y=w270:dbl[])
        n150 = call-poly <vilib>:"Mean.vi"("X"=w270) -> ("mean"=w269:dbl)  [unwired: 1 out]
      }
      n151 = call-poly <vilib>:"Mean.vi"("X"=w235) -> ()  [unwired: 2 out]
      n152 = call "Std Deviation and Variance.vi"("X"=w239) -> ()  [unwired: 1 in, 3 out]
    }
    frame "Mean Trace" {
      w311 = 0.0 ("standard deviation")
      n153 = Unbundle By Name(w315) -> ("Data File"=w326:T7, "Impulse Positions"=w325:T8, "desaccading parameters.Impulse dir"=w324:bool, "desaccading parameters.Impulse Plane 2"=w323:T9, "desacc"=w322:T10)
      n154 = property class="Arr (strict)"(reference=w304) -> ("Value"=w320:T11)  [unwired: 1 in, 2 out]
      n155 = property class="Bool (strict)"(reference=w303) -> ("Value"=w306:bool)  [unwired: 1 in, 2 out]
      n156 = call "Couple Head Impulse Traces.vi"("Data Input"=w326, "Impulse Positions"=w325, "Trace Select"="Trace Select", "Impulse Direction +ve?"=w324, "Impulse Plane"=w323, "Mean and STD"=FALSE ("Mean Traces"), "Plot Selection 2"=w320, "desacc"=w322, "Interpolate"=w306) -> ("Impulses"=w314:dbl[][])  [unwired: 7 in, 3 out]
      n157 = Array Size(array=w320) -> (size(s)=w316:i32)
      n158 = Array Size(array=w314) -> (size(s)=w319:i32[])
      n159 = Index Array(array=w319, index=0) -> (element=w317:i32)
      n160 = Quotient & Remainder(x=w317, y=w316) -> (floor(x/y)=w313:i32)  [unwired: 1 out]
      n161 = for {
        N: w313 -> [w346]
        tunnel: [w341] -> w312 mode=indexing
        tunnel: w308 -> [w340]
        tunnel: w314 -> [w344]
        tunnel: w309 -> [w339]
        tunnel: w308 -> [w338]
        tunnel: [w336] -> w307 mode=indexing
        i -> [w345]
        n162 = Add(x=w346, y=w345) -> (x+y=w347:i32)
        n163 = Index Array(array=w344, index (row)=w345) -> (element=w337:dbl[])  [unwired: 1 in]
        n164 = Index Array(array=w344, index (row)=w347) -> (element=w343:dbl[])  [unwired: 1 in]
        n165 = Multiply(x=w340, y=6.283185307179586) -> (x*y=w348:dbl)
        n166 = for {
          tunnel: w348 -> [w362]
          tunnel: [w355] -> w349 mode=indexing
          tunnel: w343 -> [_] mode=indexing
          i -> [w361]
          n167 = Multiply(x=w362, y=w361) -> (x*y=w360:dbl)
          n168 = Multiply(y=w360) -> (x*y=w359:dbl)  [unwired: 1 in]
          n169 = Cosine(x=w359) -> (cos(x)=w358:dbl)
          n170 = Sine(x=w359) -> (sin(x)=w357:dbl)
          n171 = Build Array(1.0 ("Input Element"), w357, w358) -> (w355:dbl[])
        }
        n172 = Reciprocal() -> (1/x=w332:dbl)  [unwired: 1 in]
        n173 = call "Remove NaNs.vi"("Sinusoid"=w349, "Response"=w343, "Stimulus"=w337) -> ("Response (out)"=w333:dbl[], "Stimulus (out)"=w335:dbl[])  [unwired: 1 out]
        n174 = case shown="True" w339 {
          tunnel: [w351 w352] -> w336
          tunnel: w338 -> [w351 _]
          tunnel: w337 -> [_ w354]
          tunnel: w332 -> [_ w353]
          frame False {
          }
          frame True {
            n175 = call "Determine Frequency.vi"("Sample Rate"=w353, "Signal (in)"=w354) -> ("Fundamental frequency"=w352:dbl)  [unwired: 5 in]
          }
        }
        n176 = Build Array(w335, w333) -> (w334:dbl[][])
        n177 = call "Differentiate 3D.vi"("Sample Rate 4"=w332, "Data (in)"=w334) -> ("Data (differentiated)"=w330:dbl[][])  [unwired: 3 in]
        n178 = Index Array(array=w330, index (row)=1) -> (element=w328:dbl[])  [unwired: 1 in]
        n179 = Index Array(array=w330, index (row)=0) -> (element=w327:dbl[])  [unwired: 1 in]
        n180 = Divide(x=w328, y=w327) -> (x/y=w342:dbl[])
        n181 = call-poly <vilib>:"Mean.vi"("X"=w342) -> ("mean"=w341:dbl)  [unwired: 1 out]
      }
      n182 = call-poly <vilib>:"Mean.vi"("X"=w307) -> ()  [unwired: 2 out]
      n183 = call "Std Deviation and Variance.vi"("X"=w312) -> ()  [unwired: 1 in, 3 out]
      n184 = Divide(x=w311, y=w311) -> ()  [unwired: 1 out]
    }
  }
  n185 = case shown="True" w12 {
    tunnel: "Cluster in" -> [w367 w369]
    tunnel: [w366 w368] -> w11
    tunnel: w4 -> [w365 _]
    tunnel: w3 -> [w364 _]
    tunnel: w2 -> [w363 _]
    frame True {
      n186 = Bundle By Name(cluster=w367, "Sinusoidal Fit Controls.Sinusoidal Stimulus"=w365, "Sinusoidal Fit Controls.Sinusoidal Response"=w364, "Sinusoidal Fit Controls.Gain and Phase"=w363) -> (w366:T1)
    }
    frame False {
      n187 = Bundle By Name(cluster=w369) -> (w368:T1)  [unwired: 2 in]
    }
  }
  "Cluster out" <- w11
